vi "Write configuration.vi"(8 "error in (no error)":errorcluster, 10 "configuration":refnum<class "CEF_serializable configuration.lvclass">, 11 "Abstract Scope":refnum<class "Scope Instrument.lvclass">) -> (0 "error out":errorcluster, 3 "Abstract Scope out":refnum<class "Scope Instrument.lvclass">)   [LabVIEW 2025, in "Scope.lvlib" / "Scope Instrument.lvclass"]
uses:
  Scope Instrument.lvclass
  Users/Public/Documents/Sandia National Labs/TSS Plugin/CEF.lvlibp/serializable configuration/CEF_serializable configuration.lvclass
  Scope configuration/Scope configuration.lvclass
  Scope Instrument.lvclass/Scope Instrument.ctl
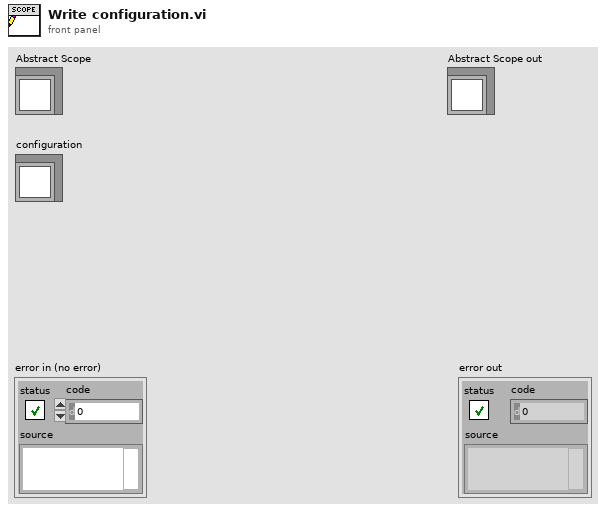
[diagram p1: front panel]
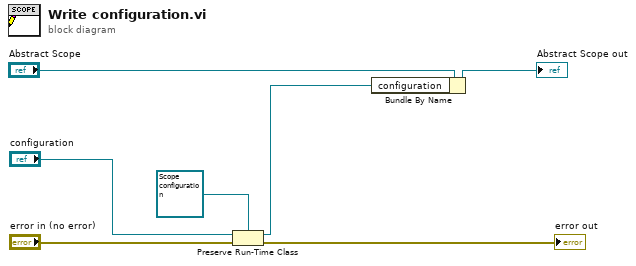
[diagram p0: block diagram]
diagram:
  n1 = Preserve Run-Time Class(object in="configuration", error in="error in (no error)", 2:refnum<class "Scope configuration.lvclass"> refnum ("Scope.lvlib:Scope configuration.lvclass")) -> (object out=w4:refnum<class "Scope configuration.lvclass">, error out=→"error out":errorcluster)
  n2 = Bundle By Name(cluster="Abstract Scope", "configuration"=w4) -> (→"Abstract Scope out":refnum<class "Scope Instrument.lvclass">)
